vi "DISP_WIND_ANN_MARK_SI_E.vi"(0 "VISA IN":refnum<visa-resource-name>, 1 "Size":string(combo)="NORM", 5 "error in":errorcluster, 7 "Window":i32) -> (14 "VISA Out":refnum<visa-resource-name>, 19 "error out":errorcluster)   [LabVIEW 2018, in "PNA-X.lvlib"]
doc: "DISPlay:WINDow<wnum>:ANNotation:MARKer:SIZE <char> \n(Read-Write) Specifies the size of the marker readout text. See other SCPI Marker commands. Learn \nmore about Marker readout. \nParameters \n<wnum> Any existing window number. If unspecified, value is set to 1. \n<char> Readout text size. Choose from:NORMal | LARGe \nExamples DISP:WIND:ANN:MARK:SIZE LARG \ndisplay:window:annotation:marker:size normal \nQuery Syntax DISPlay:WINDow:ANNotation:MARKer:SIZE? \nReturn Type Character \nDefault NORMal \n1590"
uses:
  PNA-X.lvlib
panel:
  in  "Cmdline":string="DISPlay:WINDow%d:ANNotation:MARKer:SIZE %s "
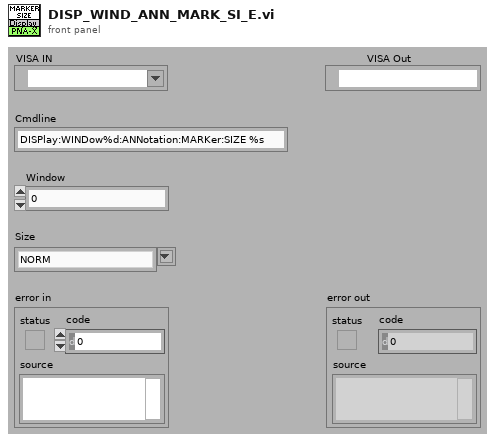
[diagram p1: front panel]
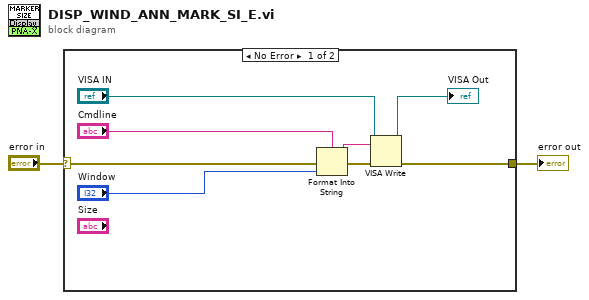
[diagram p0: block diagram]
diagram:
  n1 = case shown="No Error" "error in" {
    selector: "error in" -> [w10 w11]
    tunnel: [w5 w11] -> w1
    frame No Error {
      n2 = Format Into String(format string="Cmdline", error in=w10, "Window") -> (resulting string=w8:string, error out=w9:errorcluster)  [unwired: 1 in]
      n3 = VISA Write(VISA resource name="VISA IN", write buffer=w8, error in (no error)=w9) -> (VISA resource name out=→"VISA Out":refnum<visa-resource-name>, error out=w5:errorcluster)  [unwired: 1 out]
    }
    frame Error {
    }
  }
  "error out" <- w1
